vi "ADIS16448_RoboRIO_Teensy_Reset.vi"(8 "error in":errorcluster, 11 "SerialPortRef":T1) -> (0 "error out":errorcluster, 3 "SerialPortRefOut":T1)   [LabVIEW 2016, in "ADIS16448-Teensy.lvlib"]
uses:
  ADIS16448-Teensy.lvlib
  <vilib>/Rock Robotics/WPI/SerialPort/WPI_SerialPortRef.ctl
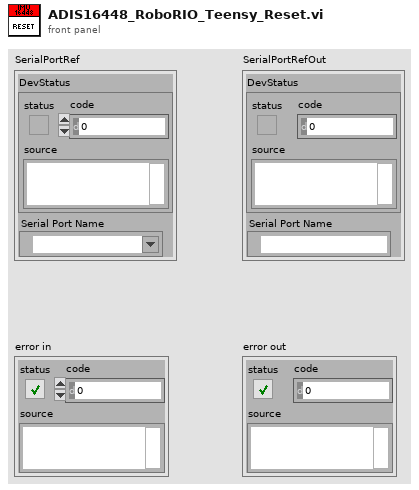
[diagram p1: front panel]
types:
  T1 = typedef "WPI_SerialPortRef.ctl" = cluster{"DevStatus":errorcluster, "Serial Port Name":refnum<visa-resource-name>}
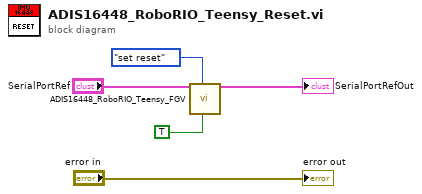
[diagram p0: block diagram]
diagram:
  n1 = call "ADIS16448_RoboRIO_Teensy_FGV.vi"("SerialPortRefIn"="SerialPortRef", "Operation"=enum16{"set", "get", "set reset"}."set reset", "Reset"=TRUE) -> ("SerialPortRefOut"=→"SerialPortRefOut":T1)  [unwired: 10 in, 6 out]
  "error out" <- "error in"
